vi "0_PTLF_Classification_Dataset_Generation.vi"() -> ()   [LabVIEW 2020]
panel:
  in  "Normalization Factor":sgl=400.0 format="%_4g"
  in  "Test Dataset size (Per Class)":i32=200
  in  "Train Dataset size (Per Class)":i32=5000
  in  "Test Dataset Folder Path":path=path "D:/Ngene/GitHub/deepltk_fpga_examples/3_PTLF_Classification(PXI,sbRIO)/Dataset/Test"
  in  "Train Dataset Folder Path":path=path "D:/Ngene/GitHub/deepltk_fpga_examples/3_PTLF_Classification(PXI,sbRIO)/Dataset/Train"
  # "Overview: This VI generates synthetic test and train datasets.\n\nInstructions:\n1. Define the sizes for the training and testing datasets for each class.\n2. Specify the location where the synthetic dataset should be stored.\n3. Execute the VI.\n4. Navigate to the paths to observe the generated datasets."
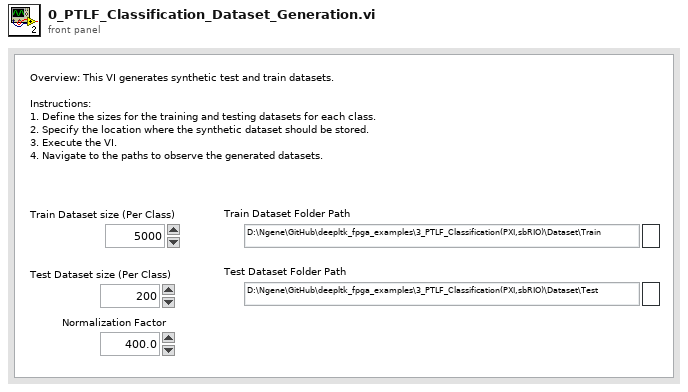
[diagram p1: front panel]
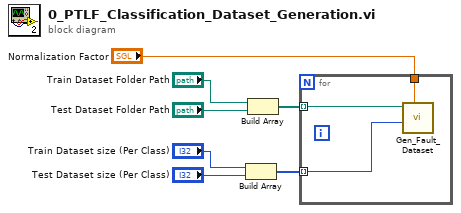
[diagram p0: block diagram]
diagram:
  n1 = Build Array("Train Dataset size (Per Class)", "Test Dataset size (Per Class)") -> (w3:i32[])
  n2 = Build Array("Train Dataset Folder Path", "Test Dataset Folder Path") -> (w5:path[])
  n3 = for {
    tunnel: w5 -> [w10] mode=indexing
    tunnel: w3 -> [w9] mode=indexing
    tunnel: "Normalization Factor" -> [w8]
    n4 = call "Gen_Fault_Dataset.vi"("Norm fctor"=w8, "Number of Samples Per Class"=w9, "Dataset Folder Path"=w10) -> ()  [unwired: 8 in, 1 out]
  }
